vi "Create New Handler.File.vi"(7 "Handler.File in":refnum<class "Handler.File.lvclass">, 8 "error in (no error)":errorcluster, 9 "File Path":path, 10 "Name":string, 11 "Level":T1(ring)) -> (0 "error out":errorcluster, 3 "Handler.File out":refnum<class "Handler.File.lvclass">)   [LabVIEW 2017, in "Error Log.lvlib" / "Handler.File.lvclass"]
uses:
  Handler.File.lvclass
  \\192.168.1.40\Neosoft/Partage/Dossiers Personnels/BRO/DevTools_BR/wc/ErrorLog/src/Handler/Handler.lvclass
  Handler.File.lvclass/Handler.File.ctl
  Handler/Handler.lvclass
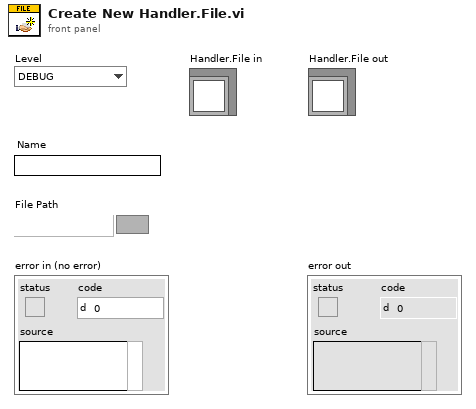
[diagram p1: front panel]
types:
  T1 = enum16{"DEBUG", "INFO", "WARNING", "ERROR", "CRITICAL"}
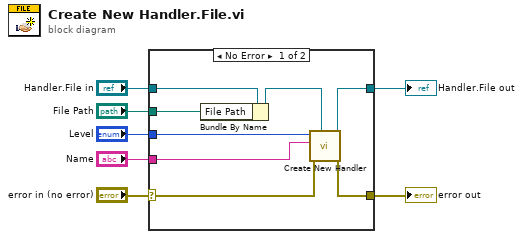
[diagram p0: block diagram]
diagram:
  n1 = case shown="No Error" "error in (no error)" {
    selector: "error in (no error)" -> [w12 w17]
    tunnel: [w11 w17] -> w6
    tunnel: [w10 w16] -> w4
    tunnel: "Handler.File in" -> [w15 w16]
    tunnel: "Level" -> [w14 _]
    tunnel: "Name" -> [w13 _]
    tunnel: "File Path" -> [w8 _]
    frame No Error {
      n2 = Bundle By Name(cluster=w15, "File Path"=w8) -> (w9:refnum<class "Handler.File.lvclass">)
      n3 = call "Create New Handler.vi"("Handler type"=w9, "error in (no error)"=w12, "Name"=w13, "Level"=w14) -> ("error out"=w11:errorcluster, "Handler"=w10:refnum<class "Handler.File.lvclass">)  [unwired: 6 in]
    }
    frame Error {
    }
  }
  "error out" <- w6
  "Handler.File out" <- w4
